vi "String to Segments.vi"(7 "Separator (dot)":string, 10 "String":string) -> (2 "Segments":string[](array[string]), 3 "Nb segments":i32)   [LabVIEW 2013, in "OpenConvert.lvlib"]
uses:
  OpenConvert.lvlib
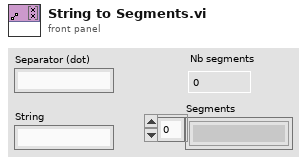
[diagram p1: front panel]
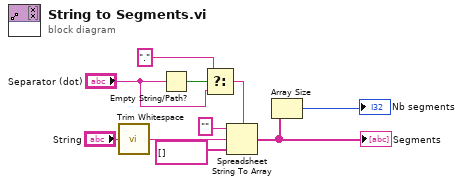
[diagram p0: block diagram]
diagram:
  n1 = call <vilib>:"Trim Whitespace.vi"("string"="String") -> ("trimmed string"=w10:string)  [unwired: 1 in]
  n2 = Empty String/Path?(string/path="Separator (dot)") -> (empty?=w7:bool)
  n3 = Select(t="." ("delimiter (Tab)"), s=w7, f="Separator (dot)") -> (s? t:f=w8:string)
  n4 = Spreadsheet String To Array(delimiter (Tab)=w8, format string="", spreadsheet string=w10, array type (2D Dbl)=string[] [] ("array")) -> (array=w2:string[])
  "Segments" <- w2
  n5 = Array Size(array=w2) -> (size(s)=→"Nb segments":i32)
